vi "PPMS Monitor.vi"(11 "IP Address":string="130.49.180.87") -> (0 "Field Graph":cluster{"X":dbl[], "Y":dbl[]}[](graph), 1 "Field (Oe)":dbl=-0.001072365790605545, 2 "Temperature Graph":cluster{"X":dbl[], "Y":dbl[]}[](graph), 3 "Temperature(K)":dbl=309.9967 format="%#_5g")   [LabVIEW 2013]
doc: "This VI monitors the PPMS temperature and magnetic field using QD Labview interface. These values are continuously updated to a global variable."
uses:
  Lock-in Globals Multiple Inputs and Outputs.vi
  PPMS Global.vi
panel:
  out "Position":dbl=-0.001072365790605545
  in  "Stop":bool
  out "Temperature Status":i32(ring)=1 items=["TemperatureUnknown"=0, "Stable"=1, "Tracking"=2, "Near"=5, "Chasing"=6, "Filling"=7, "Standby"=10, "Disabled"=13, "ImpedanceNotFunction"=14, "TempFailure"=15]
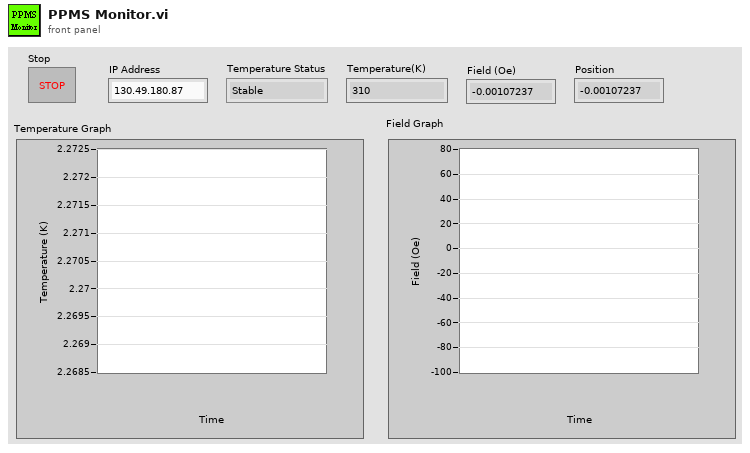
[diagram p1: front panel]
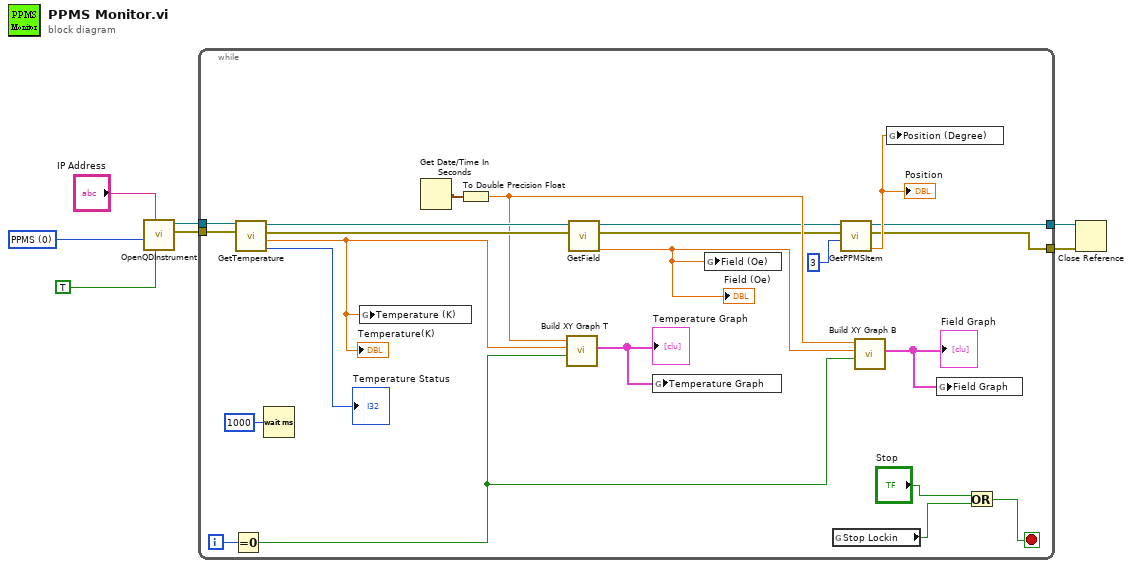
[diagram p0: block diagram]
diagram:
  w5 = 0 items=["PPMS", "VersaLab", "DynaCool", "SVSM"] ("Instrument\nType")
  n1 = call "OpenQDInstrument.vi"("Remote"=TRUE, "IP Address"="IP Address", "Instrument Type"=w5) -> ("error out"=w3:errorcluster, "Instrument Ref"=w4:refnum<k24>)  [unwired: 5 in]
  n2 = while {
    tunnel: w4 -> [w30]
    tunnel: w3 -> [w29]
    tunnel: [w9] -> w2
    tunnel: [w8] -> w1
    i -> [w25]
    stop <- w18 stop-if-true
    n3 = Equal To 0?(x=w25) -> (x = 0?=w21:bool)
    n4 = call "GetTemperature.vi"("error in (no error)"=w29, "Instrument Ref In"=w30) -> ("Temperature\nStatus"=→"Temperature Status":i32, "Temperature"=w16:dbl, "error out"=w24:errorcluster, "Instrument Ref Out"=w23:refnum<k24>)  [unwired: 3 in, 1 out]
    "Temperature(K)" <- w16
    n5 = Wait (ms)(milliseconds to wait=u32 1000) -> ()  [unwired: 1 out]
    n6 = global write "PPMS Global.vi" "Temperature (K)"(w16) -> ()
    n7 = Get Date/Time In Seconds() -> (seconds since 1Jan1904=w26:timestamp)
    n8 = To Double Precision Float(number=w26) -> (double precision float=w22:dbl)
    n9 = call "Build XY Graph T"("Reset"=w21, "Y Input"=w16, "X Input"=w22) -> ("XY Graph"=w14:cluster{"X":dbl[], "Y":dbl[]}[])  [unwired: 7 in, 1 out]
    "Temperature Graph" <- w14
    n10 = call "GetField.vi"("error in (no error)"=w24, "Instrument Ref In"=w23) -> ("Field"=w17:dbl, "error out"=w11:errorcluster, "Instrument Ref Out"=w12:refnum<k24>)  [unwired: 3 in, 2 out]
    "Field (Oe)" <- w17
    n11 = global write "PPMS Global.vi" "Temperature Graph"(w14) -> ()
    n12 = global write "PPMS Global.vi" "Field (Oe)"(w17) -> ()
    n13 = global read "Lock-in Globals Multiple Inputs and Outputs.vi" "Stop Lockin"() -> (w19:bool)
    n14 = call "GetPPMSItem.vi"("Channel"=3, "error in (no error)"=w11, "Instrument Ref In"=w12) -> ("Result"=w10:dbl, "error out"=w8:errorcluster, "Instrument Ref Out"=w9:refnum<k24>)  [unwired: 1 in, 1 out]
    "Position" <- w10
    n15 = call "Build XY Graph B"("Reset"=w21, "Y Input"=w17, "X Input"=w22) -> ("XY Graph"=w15:cluster{"X":dbl[], "Y":dbl[]}[])  [unwired: 7 in, 1 out]
    "Field Graph" <- w15
    n16 = global write "PPMS Global.vi" "Position (Degree)"(w10) -> ()
    n17 = global write "PPMS Global.vi" "Field Graph"(w15) -> ()
    n18 = Or(x="Stop", y=w19) -> (x .or. y?=w18:bool)
  }
  n19 = Close Reference(reference=w2, error in (no error)=w1) -> ()  [unwired: 1 out]
